vi "TrackExistingFaces.vi"(8 "error in (no error)":errorcluster, 9 "Image in":T1, 10 "Check face":bool, 11 "Refnum in":T2) -> (0 "error out":errorcluster, 1 "Array":T3[](array[typedef]) {"Rotation" format="%.2f"; "Left" scale=0.0..1024.0; "Right" scale=0.0..1024.0}, 2 "Image (duplicate)":T1, 3 "Refnum out":T2)   [LabVIEW 2019]
uses:
  <vilib>/vision/Tracking.llb/IMAQ Object Tracking Session.ctl
  <vilib>/vision/Image Controls.llb/IMAQ Image.ctl
  <vilib>/vision/NI_Vision_Development_Module.lvlib
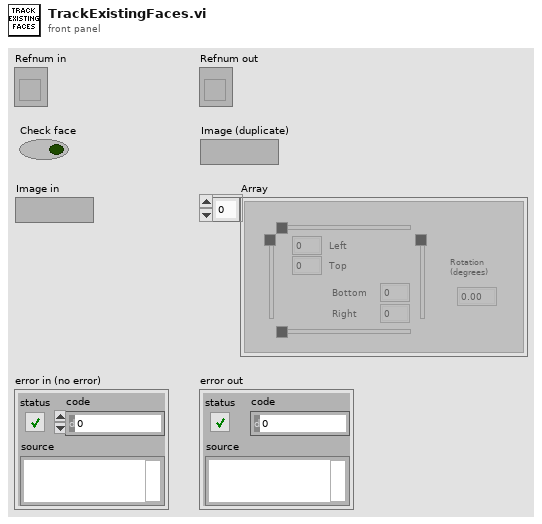
[diagram p1: front panel]
types:
  T1 = typedef "IMAQ Image.ctl" = refnum<image>
  T2 = typedef "IMAQ Object Tracking Session.ctl" = refnum<k20>
  T3 = typedef "IMAQ Rectangle" = cluster{"Left":i32, "Top":i32, "Right":i32, "Bottom":i32, "Rotation":dbl}
  T4 = cluster{"Label":string, "Score":i32, "Angle":dbl, "Location":cluster{"X":dbl, "Y":dbl}, "Bounding Box":cluster{"X":dbl, "Y":dbl}[], "Object Found?":bool}[]
  T5 = typedef "Image Type" = u32
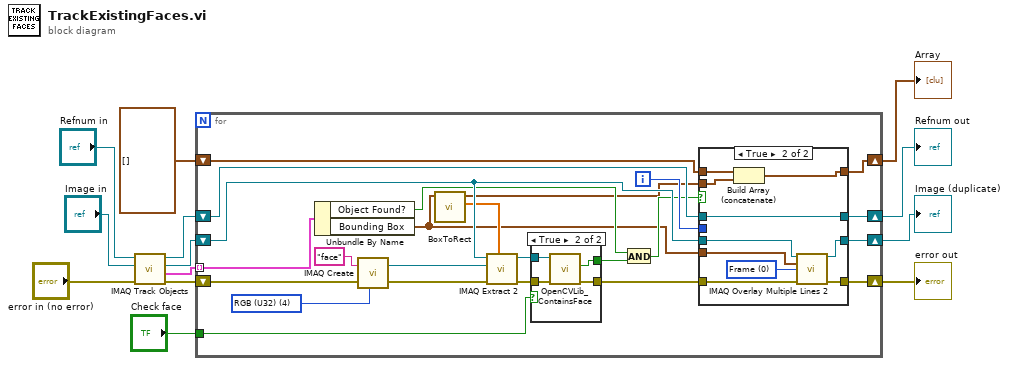
[diagram p0: block diagram]
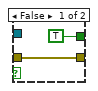
[diagram p2: hidden frame]
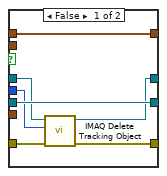
[diagram p3: hidden frame]
diagram:
  n1 = call "IMAQ Track Objects"("error in (no error)"="error in (no error)", "Image"="Image in", "Object Tracking Session In"="Refnum in") -> ("error out"=w2:errorcluster, "Objects (pixel)"=w8:T4, "Image (duplicate)"=w1:T1, "Object Tracking Session Out"=w9:T2)  [unwired: 1 in, 4 out]
  n2 = for {
    shift-right: [w35] -> w7
    shift-left: w1 -> [w28]
    shift-right: [w37] -> w6
    shift-left: w2 -> [w25]
    tunnel: w8 -> [w36] mode=indexing
    shift-right: [w32] -> w10
    shift-left: w9 -> [w33]
    shift-right: [w21] -> w11
    shift-left: T3[] [] -> [w31]
    tunnel: "Check face" -> [w18]
    i -> [w34]
    w20 = T5 4 items=["Grayscale (U8)", "Grayscale (I16)", "Grayscale (SGL)", "Complex (CSG)", "RGB (U32)", "HSL (U32)", "RGB (U64)", "Grayscale (U16)"] ("Image Type")
    n3 = Unbundle By Name(w36) -> ("Object Found?"=w24:bool, "Bounding Box"=w19:cluster{"X":dbl, "Y":dbl}[])
    n4 = call "IMAQ Create"("Image Name"="face", "Image Type"=w20, "error in (no error)"=w25) -> ("New Image"=w29:T1, "error out"=w26:errorcluster)  [unwired: 2 in]
    n5 = call "BoxToRect.vi"("Bounding Box"=w19) -> ("Array"=w27:dbl[], "Rectangle"=w22:T3)  [unwired: 9 in]
    n6 = call "IMAQ Extract 2"("Optional Rectangle"=w27, "error in (no error)"=w26, "Image Dst"=w29, "Image Src"=w28) -> ("error out"=w17:errorcluster, "Image Dst Out"=w16:T1)  [unwired: 6 in]
    n7 = case shown="True" w18 {
      tunnel: w17 -> [w38 w43]
      tunnel: w16 -> [_ w42]
      tunnel: [w38 w41] -> w15
      tunnel: [TRUE ("Contrains Face") w40] -> w14
      frame False {
      }
      frame True {
        n8 = call "OpenCVLib_ContainsFace.vi"("error in (no error)"=w43, "Image Src"=w42) -> ("error out"=w41:errorcluster, "Contrains Face"=w40:bool)  [unwired: 7 in, 1 out]
      }
    }
    n9 = And(x=w24, y=w14) -> (x .and. y?=w23:bool)
    n10 = case shown="True" w23 {
      tunnel: w28 -> [w50 w54]
      tunnel: [w50 w56] -> w35
      tunnel: w15 -> [w48 w57]
      tunnel: [w47 w55] -> w37
      tunnel: w34 -> [w49 _]
      tunnel: w33 -> [w46 w60]
      tunnel: [w45 w60] -> w32
      tunnel: [w44 w59] -> w21
      tunnel: w31 -> [w44 w58]
      tunnel: w22 -> [_ w53]
      tunnel: w19 -> [_ w52]
      frame False {
        n11 = call "IMAQ Delete Tracking Object"("error in (no error)"=w48, "Object Index"=w49, "Object Tracking Session In"=w46) -> ("error out"=w47:errorcluster, "Object Tracking Session Out"=w45:T2)  [unwired: 7 in]
      }
      frame True {
        w51 = u32 0 items=["Frame", "Fill"] ("Drawing Mode (Frame)")
        n12 = Build Array (concatenate)(w58, w53) -> (w59:T3[])
        n13 = call "IMAQ Overlay Multiple Lines 2"("Image"=w54, "Line End Points"=w52, "Drawing Mode (Frame)"=w51, "error in (no error)"=w57) -> ("Image Out"=w56:T1, "error out"=w55:errorcluster)  [unwired: 10 in]
      }
    }
  }
  "Array" <- w11
  "Refnum out" <- w10
  "Image (duplicate)" <- w7
  "error out" <- w6
